vi "OpenCycle.vi"(0 "PLC":refnum<vi>) -> ()   [LabVIEW 2023]
uses:
  S7Plc.ctl
  D:/Projects/S7View/S7Lib/bin/Debug/S7.Net.dll
  S7Lib/bin/Debug/S7.Net.dll
  D:/Projects/S7View/S7Lib/bin/Debug/S7Lib.dll
  S7Lib/bin/Debug/S7Lib.dll
panel:
  out "S7PLC":T1={"ip"="192.168.10.10", "type"=40, "rack"=0, "slot"=0, "status"=FALSE, "link"=FALSE, "msg"="", "plc"=refnum} {"type" items=["S7200"=0, "Logo0BA8"=1, "S7200Smart"=2, "S7300"=10, "S7400"=20, "S71200"=30, "S71500"=40]}
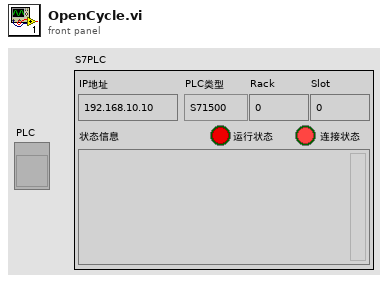
[diagram p1: front panel]
types:
  T1 = typedef "S7Plc.ctl" = cluster{"ip":string, "type":i16, "rack":i16, "slot":i16, "status":bool, "link":bool, "msg":string, "plc":refnum<k24>}
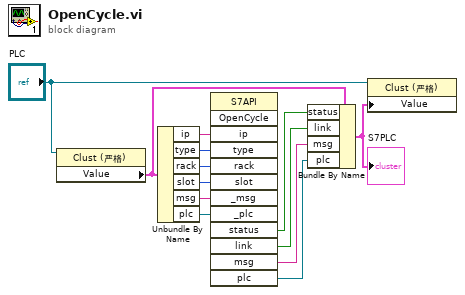
[diagram p0: block diagram]
diagram:
  n1 = property on="属性节点" class="Clust (严格)"(reference="PLC") -> ("Value"=w6:T1)  [unwired: 1 in, 2 out]
  n2 = Unbundle By Name(w6) -> ("ip"=w13:string, "type"=w12:i16, "rack"=w11:i16, "slot"=w10:i16, "msg"=w5:string, "plc"=w4:refnum<k24>)
  n3 = invoke on="调用节点" class="S7API" method="OpenCycle"("ip"=w13, "type"=w12, "rack"=w11, "slot"=w10, "_msg"=w5, "_plc"=w4) -> ("status"=w9:bool, "link"=w8:bool, "msg"=w3:string, "plc"=w7:refnum<k24>)  [unwired: 7 in, 9 out]
  n4 = Bundle By Name(cluster=w6, "status"=w9, "link"=w8, "msg"=w3, "plc"=w7) -> (w2:T1)
  "S7PLC" <- w2
  n5 = property on="属性节点" class="Clust (严格)"(reference="PLC", "Value"=w2) -> ()  [unwired: 1 in, 2 out]
